vi "SetStepFrequency.vi"(0 "handle in":i32, 1 "UnitAddress(0)":u16, 5 "error in(no error)":errorcluster, 7 "ClockDivider (5)":u8=5) -> (14 "handle out":i32, 19 "error out":errorcluster)   [LabVIEW 2014, in "Sixpack - Driver.lvlib"]
doc: "ACHTUNG: Einstellung gilt für alle Motoren gemeinsam, nur bei stehenden Motoren ändern!\n\nSetzt die Variable ClockDivider, den Vorteiler für die Schrittfrequenzberechnung fest. Dieser Wert gilt für alle Motoren gemeinsam. Der achsenindividuelle Vorteiler Div wird im Befehl SetVMinVStart beschrieben. \n(siehe Manual Seite 22 Kapite 3.3 Einstellungen zur Anpassung der Schrittberechnung für den Motor)"
uses:
  Sixpack - Driver.lvlib
  DLL/PackDLL.dll
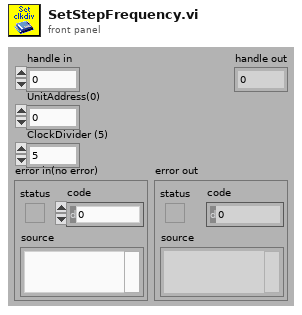
[diagram p1: front panel]
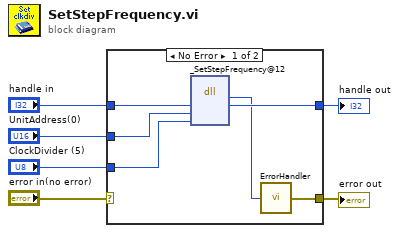
[diagram p0: block diagram]
diagram:
  n1 = case shown="No Error" "error in(no error)" {
    selector: "error in(no error)" -> [_ w14]
    tunnel: "handle in" -> [w12 w13]
    tunnel: [w11 w13] -> w5
    tunnel: "UnitAddress(0)" -> [w10 _]
    tunnel: "ClockDivider (5)" -> [w9 _]
    tunnel: [w7 w14] -> w2
    frame No Error {
      n2 = dll-call lib="D:/CS-Source/LV2014/GPL/instr.lib/SixPack/PackDLL/DLL/PackDLL.dll" fn="_SetStepFrequency@12" label="SetStepFrequency"("HANDLE"=w12, "UnitAddress"=w10, "ClockDivider"=w9) -> ("BOOLEAN"=w8:i8, "HANDLE"=w11:i32)  [unwired: 5 in, 2 out]
      n3 = call "ErrorHandler.vi"("BOOLEAN"=w8) -> ("error out"=w7:errorcluster)
    }
    frame Error {
    }
  }
  "handle out" <- w5
  "error out" <- w2
